vi "MT Close Session.vi"(0 "modulation session":T1, 11 "error in (no error)":errorcluster) -> (15 "error out":errorcluster)   [LabVIEW 2020, in "niDMT.lvlib"]
doc: "Closes any open modulation session."
uses:
  <vilib>/addons/Modulation/niDMT.lvlib
  <vilib>/addons/Modulation/Digital/Support/Controls/MT Generic Refnum.ctl
  NIMTAttribs.dll
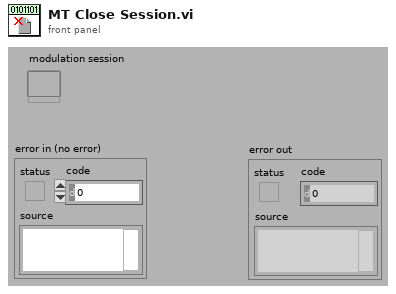
[diagram p1: front panel]
types:
  T1 = typedef "niDMT.lvlib/MT Generic Refnum.ctl" = refnum<k20>
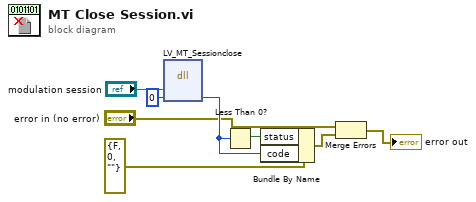
[diagram p0: block diagram]
diagram:
  n1 = dll-call lib="NIMTAttribs.*" fn="LV_MT_Sessionclose"("refnum"="modulation session", "error"=0) -> ("error"=w4:i32)  [unwired: 4 in, 3 out]
  n2 = Less Than 0?(x=w4) -> (x < 0?=w5:bool)
  n3 = Bundle By Name(cluster=errorcluster {"status"=FALSE, "code"=0, "source"=""} ("error in (no error) 2"), "status"=w5, "code"=w4) -> (w2:errorcluster)
  n4 = Merge Errors("error in (no error)", w2) -> (→"error out":errorcluster)
